vi "LimitedRead.vi"(3 "MaxTime":u32, 4 "MaxLength":u8, 5 "ReadFIFO":refnum<k21>, 6 "OutFIFO":refnum<k21>) -> (0 "Timedout":u8, 2 "ReadBytes":i16)   [LabVIEW 2023]
uses:
  <vilib>/Platform/TimedLoop/XDataNode/timing_clust.ctl
  <vilib>/Platform/TimedLoop/XDataNode/nitl_modes.ctl
  <vilib>/Platform/TimedLoop/XDataNode/wakeup.ctl
  <vilib>/rvi/Emulation/niFpgaSctlEmulationGetInTimedLoop.vi
  <vilib>/rvi/Emulation/niFpgaEmulationReportErrorSimple.vi
  <vilib>/rvi/Emulation/niFpgaGetClockAttributes.vi
  <vilib>/rvi/Emulation/niFpgaCriticalErrorInLSC.vi
  <vilib>/rvi/DataTransferAndStorage/Container/Common/niFpgaContainerExecOnDevCompGetState.vi
  <vilib>/rvi/Emulation/niFpgaEmulationIsFPGAContextNoSignature.vi
  <vilib>/rvi/errors/niFpgaSetErrorForExecOnDevCompSimple.vi
  <vilib>/rvi/eio/common/nirviEmuReportErrorAndStop.vi
  <vilib>/rvi/DataTransferAndStorage/Container/Common/niFpgaContainerGetUniqueNameForEmu.vi
  <vilib>/rvi/FIFO/Fifo_Resource/nirvififoEmulationSetSize.vi
  <vilib>/rvi/FIFO/Fifo_Resource/nirviFifoEmulationQueueMgr.vi
  <instcachedir>/0/nirviFifoEmulationQueueMgr_E5CAEC123FF24DC58D834DCA3CDAA9B5.lvgen/nirviFifoEmulationQueueMgr_E5CAEC123FF24DC58D834DCA3CDAA9B5_002.vi
  <vilib>/rvi/FIFO/Fifo_Resource/nirvififoEmulationDetermineInputValidOut.vi
  <vilib>/rvi/FIFO/Fifo_Resource/nirvififoEmulationCreateLock.vi
  <vilib>/rvi/Emulation/niFpgaProcessEmulError.vi
  <vilib>/rvi/FIFO/Fifo_Resource/nirvififoEmulationObtainLock.vi
  <vilib>/rvi/FIFO/Fifo_Resource/nirvififoEmulationReleaseLock.vi
  <vilib>/rvi/occurrence/nirviWaitOnOccurrenceBase.vi
  <vilib>/rvi/errors/nirviReportUnexpectedCaseInternalError.vi
  <vilib>/rvi/errors/nirviReportUnexpectedCaseInternalError (U32).vi
  <vilib>/Utility/error.llb/Clear Errors.vi
  <vilib>/eio/utilities/niEioResolveVilibRelativePath.vi
  <vilib>/rvi/interface/RandomDataEmulation/niFpgaRandomDataHandleErrors.vi
  <vilib>/Platform/TimedLoop/XDataNode/XDataNode.xnode
  <vilib>/rvi/DataTransferAndStorage/Container/XNode/niFpgaContainer.xnode
  <vilib>/rvi/FIFO/Fifo_Resource/niFpgaFifoEmulationRefIn.vi
  <vilib>/Platform/TimedLoop/XDataNode/XDNodeRunTimeDep.lvlib
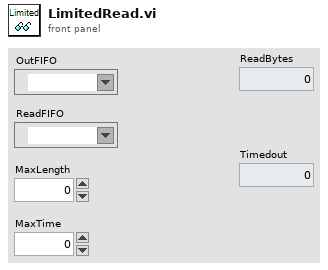
[diagram p1: front panel]
types:
  T1 = typedef "XDNodeRunTimeDep.lvlib/timing_clust.ctl" = cluster{"Expected End [f-1]":u64, "Actual End [f-1]":u64, "Finished Late? [f-1]":bool, "Expected End [i-1]":u64, "Actual End [i-1]":u64, "Finished Late? [i-1]":bool, "Expected Start [i]":u64, "Actual Start [i]":u64, "Expected Start [f]":u64, "Actual Start [f]":u64, "Source Name":string, "Structure Name":string, "Period":i64, "Deadline":i64, "Offset":i64, "Start":i64, "Priority":i32, "Timeout":i32, "Mode":T2, "Wakeup Reason":T3, "Error":errorcluster, "Source Type":string, "Secondary Source Type":string, "Global End Time":u64, "Global Start Time":u64, "Frame Duration":u64, "Iteration Duration":u64, "Assigned CPU":i32, "I/O Scan Engine Mode":u32}
  T2 = typedef "XDNodeRunTimeDep.lvlib/nitl_modes.ctl" = enum32{"No Change", "Process missed periods, maintain original phase", "Discard missed periods, maintain original phase", "Process missed periods, ignore original phase", "Discard missed periods, ignore original phase"}
  T3 = typedef "XDNodeRunTimeDep.lvlib/wakeup.ctl" = enum32{"Normal", "Aborted", "Asynchronous wakeup", "Timing source error", "Timed loop error", "Timeout"}
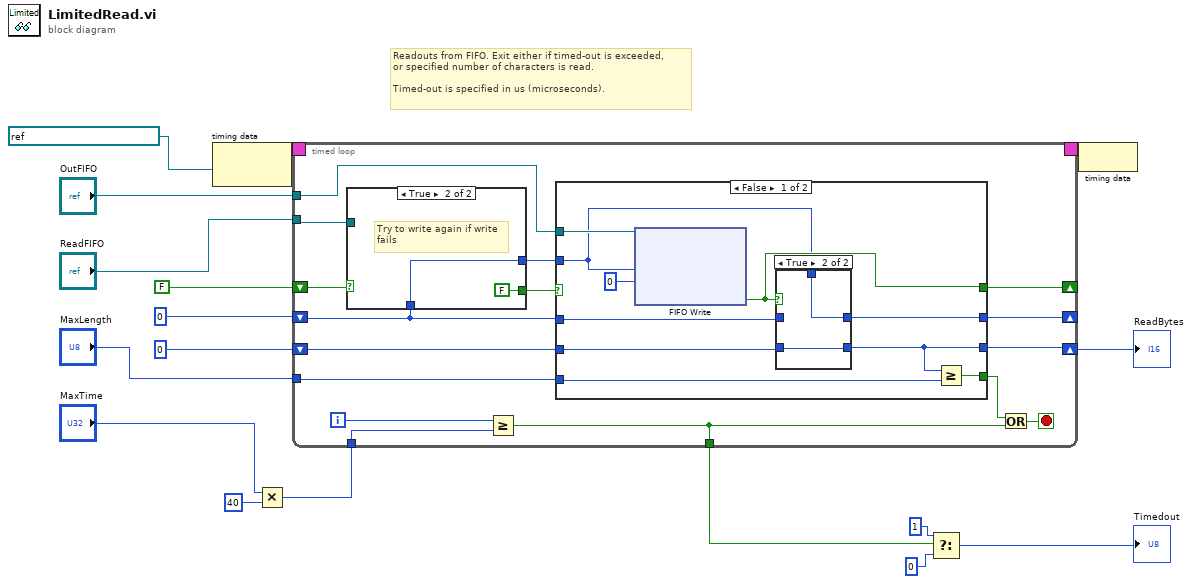
[diagram p0: block diagram]
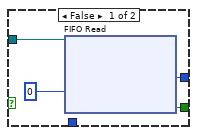
[diagram p2: hidden frame]
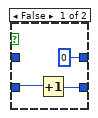
[diagram p3: hidden frame]
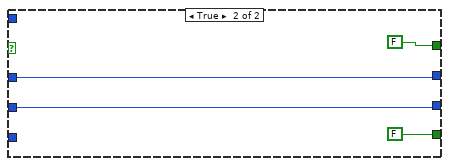
[diagram p4: hidden frame]
diagram:
  # "Readouts from FIFO. Exit either if timed-out is exceeded,\nor specified number of characters is read.\n\nTimed-out is specified in us (microseconds)."
  n1 = node-c288(refnum<k21> "40 MHz Onboard Clock" ("Source Name")) -> (w17:T1)
  n2 = Multiply(x="MaxTime", y=u32 40) -> (x*y=w9:u32)
  n3 = timed-loop {
    timing: w17 -> [_]
    timing-out: [_] -> w16
    tunnel: "ReadFIFO" -> [w33]
    tunnel: "OutFIFO" -> [w20]
    shift-right: [w21] -> w8
    shift-left: u8 0 -> [w31]
    tunnel: "MaxLength" -> [w30]
    shift-right: [w29] -> _
    shift-left: u8 0 -> [w18]
    tunnel: w9 -> [w27]
    tunnel: [w24] -> w2
    shift-right: [w22] -> _
    shift-left: FALSE -> [w19]
    i -> [w28]
    stop <- w26 stop-if-true
    n4 = case shown="True" w19 {
      tunnel: w33 -> [w37 _]
      tunnel: [w35 w39] -> w32
      tunnel: [w34 FALSE ("Timed Out?")] -> w25
      tunnel: w18 -> [_ w39]
      frame False {
        n5 = xnode ("FIFO Read")("Timeout"=0, "FIFO In"=w37) -> ("Element"=w35:u8, "Timed Out?"=w34:bool)  [unwired: 1 out]
      }
      frame True {
        # "Try to write again if write\nfails"
      }
    }
    n6 = Greater Or Equal?(x=w28, y=w27) -> (x >= y?=w24:bool)
    n7 = case shown="False" w25 {
      tunnel: w32 -> [w40 _]
      tunnel: w20 -> [w49 _]
      tunnel: w31 -> [w42 w58]
      tunnel: w30 -> [w47 _]
      tunnel: w18 -> [w46 w56]
      tunnel: [w45 w56] -> w29
      tunnel: [w44 FALSE] -> w23
      tunnel: [w41 FALSE ("Timed Out?")] -> w22
      tunnel: [w43 w58] -> w21
      frame False {
        n8 = xnode ("FIFO Write")("Element"=w40, "Timeout"=0, "FIFO In"=w49) -> ("Timed Out?"=w41:bool)  [unwired: 1 out]
        n9 = case shown="True" w41 {
          tunnel: w46 -> [_ _]
          tunnel: [u8 0 w53] -> w45
          tunnel: [w52 w54] -> w43
          tunnel: w42 -> [w51 w54]
          tunnel: w40 -> [_ w53]
          frame False {
            n10 = Increment(x=w51) -> (x+1=w52:u8)
          }
          frame True {
          }
        }
        n11 = Greater Or Equal?(x=w43, y=w47) -> (x >= y?=w44:bool)
      }
      frame True {
      }
    }
    n12 = Or(x=w23, y=w24) -> (x .or. y?=w26:bool)
  }
  "ReadBytes" <- w8
  n13 = Select(t=u8 1, s=w2, f=u8 0) -> (s? t:f=→"Timedout":u8)
  n14 = node-c288(w16) -> ()
